vi "CalExample.vi"() -> ()   [LabVIEW 2015, in "QCA_DUT_Func.lvlib"]
uses:
  QCA_DUT_Func.lvlib
  WTSInstrumentControl/PhyPort.ctl
  WTSInstrumentControl/VISAOperation.ctl
panel:
  in  "PathlossConfig":T2={"PathlossFilePath"=path "D:/4-Up-WLAN-Test-System/WTSInstrumentControl/Pathloss/External Pathloss.txt", "Pathloss Table Name"="wlan", "PhyPort"=enum."Port5"}
  in  "VISA resource name":refnum<visa-resource-name>="TCPIP0::10.144.41.48::inst0::INSTR"
  out "return type 4":i32=41
  out "return type 3":i32
  in  "XtalCalConfig":T3={"channel"=5500, "txChain0"=1, "iXtalTargetPPM"=0, "iXtalTolerancePPM"=2, "numMeasAvg"=1, "dXtalCalSaveOption"=5, "XtalCapDelta"=56, "VISA"="TCPIP0::wts::inst0::INSTR", "Port"=5}
  out "return type 2":u8=1
  out "return type":u8=1
  in  "Bin_file":string="D:\\4-Up-WLAN-Test-System\\board_data\\boardData_QCA9984_CUS239_5G_v1_001.bin"
  in  "chip_select":i32=3
  in  "DUT_IP":string="192.168.1.2"
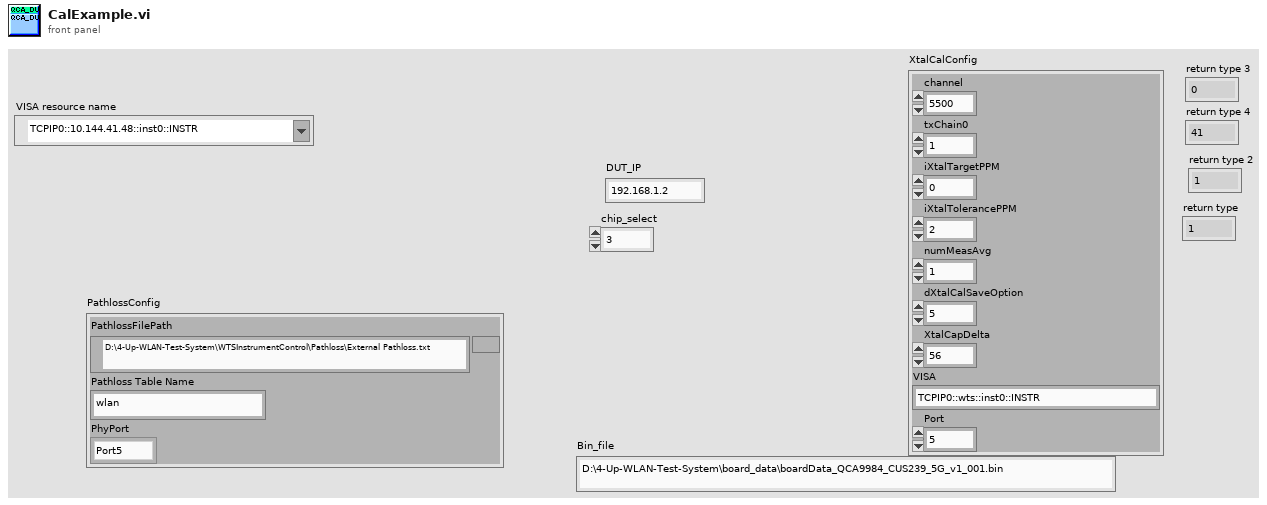
[diagram p1: front panel]
types:
  T1 = typedef "PhyPort.ctl" = enum16{"Port0", "Port1", "Port2", "Port3", "Port4", "Port5", "Port6", "Port7"}
  T2 = cluster{"PathlossFilePath":path, "Pathloss Table Name":string, "PhyPort":T1}
  T3 = cluster{"channel":i32, "txChain0":i32, "iXtalTargetPPM":i32, "iXtalTolerancePPM":u32, "numMeasAvg":u32, "dXtalCalSaveOption":u32, "XtalCapDelta":i32, "VISA":string, "Port":i32}
  T4 = typedef "VISAOperation.ctl" = enum16{"RunFile", "OpenDebugPanel", "ReadError", "ReadSTB", "Reset", "Clean", "CloseVISA", "RunCMD", "OpenVISA"}
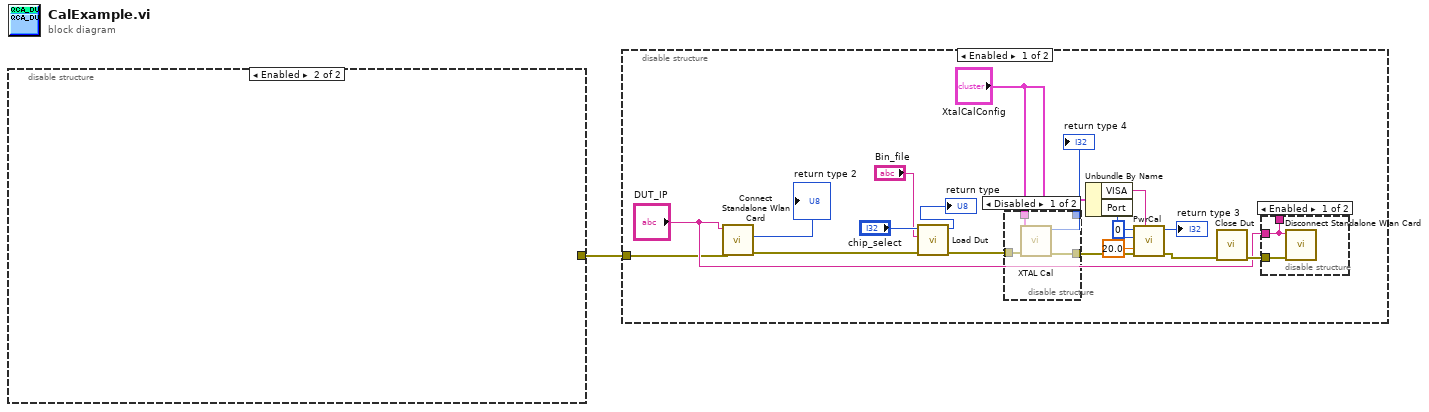
[diagram p0: block diagram]
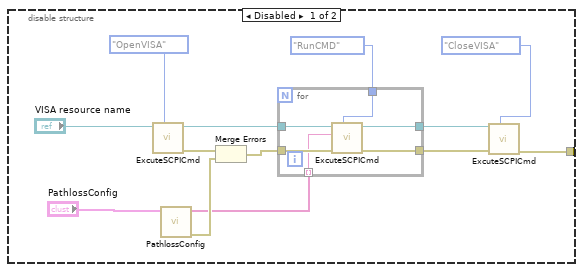
[diagram p2: hidden frame]
diagram:
  n1 = disable-structure shown="Enabled" {
    disable-tunnel: [w2 _] -> w1
    frame Disabled {
      n2 = call "ExcuteSCPICmd.vi"("VISAOperation"=VISAOperation."OpenVISA", "VISA resource name"="VISA resource name") -> ("error out"=w11:errorcluster, "reference out"=w10:refnum<visa-resource-name>)  [unwired: 6 in, 2 out]
      n3 = call "PathlossConfig.vi"("PathlossConfig"="PathlossConfig") -> ("error out"=w5:errorcluster, "PahtlossCMD"=w4:string[])  [unwired: 9 in]
      n4 = Merge Errors(w11, w5) -> (w8:errorcluster)
      n5 = for {
        tunnel: VISAOperation."RunCMD" ("VISAOperation") -> [w18]
        tunnel: w10 -> [w20]
        tunnel: [w19] -> w6
        tunnel: w8 -> [w17]
        tunnel: w4 -> [w16] mode=indexing
        tunnel: [w15] -> w3
        n6 = call "ExcuteSCPICmd.vi"("VISAOperation"=w18, "error in (no error)"=w17, "Run Command"=w16, "VISA resource name"=w20) -> ("error out"=w15:errorcluster, "reference out"=w19:refnum<visa-resource-name>)  [unwired: 4 in, 2 out]
      }
      n7 = call "ExcuteSCPICmd.vi"("VISAOperation"=VISAOperation."CloseVISA", "error in (no error)"=w3, "VISA resource name"=w6) -> ("error out"=w2:errorcluster)  [unwired: 5 in, 3 out]
    }
    frame Enabled {
    }
  }
  n8 = disable-structure shown="Enabled" {
    disable-tunnel: w1 -> [w22 _]
    frame Enabled {
      n9 = call "Connect Standalone Wlan Card.vi"("error in (no error)"=w22, "DUT_IP"="DUT_IP") -> ("error out"=w37:errorcluster, "return type"=→"return type 2":u8)  [unwired: 7 in, 1 out]
      n10 = call "Load Dut.vi"("error in (no error)"=w37, "Bin_file"="Bin_file", "chip_select"="chip_select") -> ("error out"=w32:errorcluster, "return type"=→"return type":u8)  [unwired: 6 in, 1 out]
      n11 = disable-structure shown="Disabled" {
        disable-tunnel: [w42 w43] -> w38
        disable-tunnel: w32 -> [w41 w43]
        disable-tunnel: "XtalCalConfig" -> [w40 _]
        disable-tunnel: [w39 _] -> w26
        frame Disabled {
          n12 = call "XTAL Cal.vi"("error in (no error)"=w41, "XtalCalConfig"=w40) -> ("error out"=w42:errorcluster, "return type"=w39:i32)  [unwired: 8 in]
        }
        frame Enabled {
        }
      }
      "return type 4" <- w26
      n13 = Unbundle By Name("XtalCalConfig") -> ("VISA"=w30:string, "Port"=w29:i32)
      n14 = call "PwrCal.vi"("VISA"=w30, "error in (no error)"=w38, "RL"=20.0, "Port"=w29, "type"=0) -> ("error out"=w24:errorcluster, "return type"=→"return type 3":i32)  [unwired: 5 in]
      n15 = call "Close Dut.vi"("error in (no error)"=w24) -> ("error out"=w25:errorcluster)  [unwired: 10 in]
      n16 = disable-structure shown="Enabled" {
        disable-tunnel: w25 -> [w45 _]
        disable-tunnel: [w44 _] -> _
        disable-tunnel: "DUT_IP" -> [w44 _]
        frame Enabled {
          n17 = call "Disconnect Standalone Wlan Card.vi"("error in (no error)"=w45, "DUT_IP"=w44) -> ()  [unwired: 8 in, 2 out]
        }
        frame Disabled {
        }
      }
    }
    frame Disabled {
    }
  }
